vi "pf_Extract_3D-Data.vi"(7 "Reverse? (F)":bool, 8 "error in (no error)":errorcluster, 10 "3D Data in":u8[](array[numeric]), 11 "IMAQ Session in":refnum<k11>) -> (0 "error out":errorcluster, 1 "Quality out":u8, 2 "Width out":sgl, 3 "IMAQ Session out":refnum<k11>, 5 "Peak out":sgl)   [LabVIEW 2025, in "Photonfocus_Toolkit.lvlib"]
uses:
  Photonfocus_Toolkit.lvlib
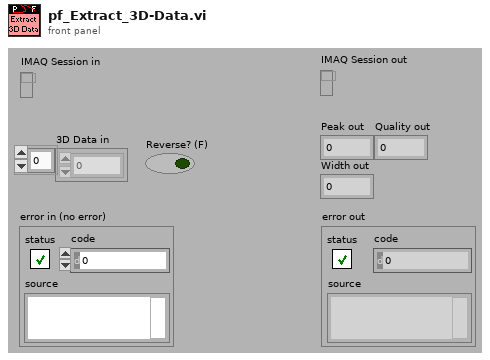
[diagram p1: front panel]
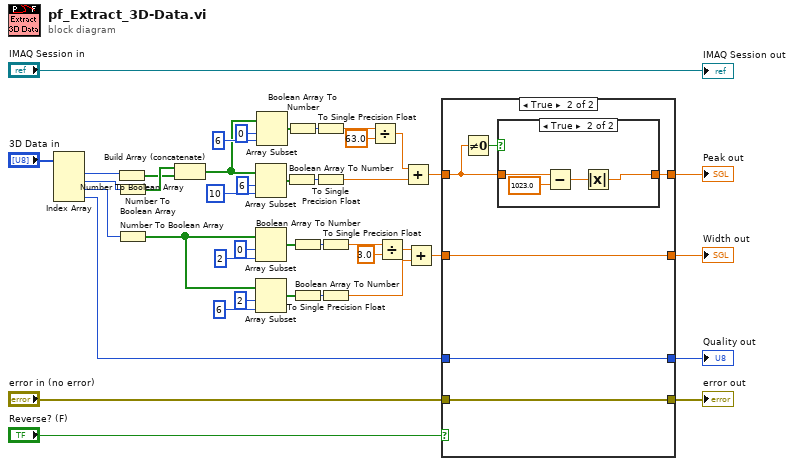
[diagram p0: block diagram]
diagram:
  n1 = Index Array(array="3D Data in") -> (element #1=w42:u8, element #2=w41:u8, element #3=w2:u8, element #4=w32:u8)  [unwired: 4 in]
  n2 = Number To Boolean Array(number=w42) -> (Boolean array=w18:bool[])
  n3 = Number To Boolean Array(number=w41) -> (Boolean array=w19:bool[])
  n4 = Number To Boolean Array(number=w2) -> (Boolean array=w8:bool[])
  n5 = Build Array (concatenate)(w19, w18) -> (w21:bool[])
  n6 = Array Subset(array=w21, index=6, length=10) -> (w26:bool[])
  n7 = Array Subset(array=w8, index=0, length=2) -> (w12:bool[])
  n8 = Array Subset(array=w8, index=2, length=6) -> (w4:bool[])
  n9 = Array Subset(array=w21, index=0, length=6) -> (w27:bool[])
  n10 = Boolean Array To Number(Boolean array=w26) -> (number=w22:u32)
  n11 = Boolean Array To Number(Boolean array=w27) -> (number=w24:u32)
  n12 = Boolean Array To Number(Boolean array=w12) -> (number=w13:u32)
  n13 = Boolean Array To Number(Boolean array=w4) -> (number=w5:u32)
  n14 = To Single Precision Float(number=w24) -> (single precision float=w17:sgl)
  n15 = To Single Precision Float(number=w22) -> (single precision float=w16:sgl)
  n16 = To Single Precision Float(number=w13) -> (single precision float=w10:sgl)
  n17 = To Single Precision Float(number=w5) -> (single precision float=w3:sgl)
  n18 = Divide(x=w17, y=sgl 63.0) -> (x/y=w23:sgl)
  n19 = Divide(x=w10, y=sgl 3.0) -> (x/y=w9:sgl)
  n20 = Add(x=w23, y=w16) -> (x+y=w20:sgl)
  n21 = Add(x=w9, y=w3) -> (x+y=w1:sgl)
  n22 = case shown="True" "Reverse? (F)" {
    tunnel: "error in (no error)" -> [w45 w49]
    tunnel: w20 -> [w46 w51]
    tunnel: [w46 w50] -> w38
    tunnel: [w45 w49] -> w37
    tunnel: w1 -> [w44 w48]
    tunnel: [w44 w48] -> w35
    tunnel: [w43 w47] -> w34
    tunnel: w32 -> [w43 w47]
    frame False {
    }
    frame True {
      n23 = Not Equal To 0?(x=w51) -> (x != 0?=w52:bool)
      n24 = case shown="True" w52 {
        tunnel: w51 -> [w53 w57]
        tunnel: [w53 w54] -> w50
        frame False {
        }
        frame True {
          n25 = Subtract(x=w57, y=sgl 1023.0) -> (x-y=w55:sgl)
          n26 = Absolute Value(x=w55) -> (abs(x)=w54:sgl)
        }
      }
    }
  }
  "Peak out" <- w38
  "error out" <- w37
  "Width out" <- w35
  "Quality out" <- w34
  "IMAQ Session out" <- "IMAQ Session in"
